vi "DJGUETTA.vi"() -> ()   [LabVIEW 2018]
uses:
  estadodjguetta.ctl
  <vilib>/myRIO/Express VI/Onboard IO/DI/DI Express VI.xnode
  <vilib>/myRIO/Instrument Drivers/Onboard IO/DIO/vis/Read.vi
  <vilib>/myRIO/Instrument Drivers/Onboard IO/DIO/DIO.lvlib
  <vilib>/myRIO/Common/Instrument Driver Framework/myRIO v1.0/DIO/typedefs/DIO Channels Enum.ctl
  <vilib>/myRIO/Common/Instrument Driver Framework/myRIO v1.0/DIO/typedefs/DIO Channels List.ctl
  <vilib>/myRIO/Common/Instrument Driver Framework/Utilities/typedefs/Generic FPGA Reference.ctl
  <vilib>/myRIO/Common/Instrument Driver Framework/Utilities/typedefs/myRIO v1.0 Reference.ctl
  <vilib>/myRIO/Common/Instrument Driver Framework/Utilities/typedefs/Hardware Version Enum.ctl
  <vilib>/myRIO/Common/Instrument Driver Framework/Utilities/typedefs/myRIO Generic Hardware Reference.ctl
  <vilib>/myRIO/Instrument Drivers/Onboard IO/DIO/typedefs/DIO Reference.ctl
  <vilib>/myRIO/Instrument Drivers/Onboard IO/DIO/vis/myRIO DIO Open.xnode
  <vilib>/myRIO/Common/Instrument Driver Framework/Utilities/vis/Is FPGA Ref Available.vi
  <vilib>/myRIO/Common/Instrument Driver Framework/myRIO v1.0/DIO/vis/myRIO v1.1 Open DIO.vi
  <vilib>/userdefined/High Color/nirio_resource_hc.ctl
panel:
  out "discos":i32
  out "yf":i32
  out "xf":i32
  out "Discos colocados":i32[](array[numeric])
  in  "Pieza":i32(slide) scale=0.0..2.0
  out "PteVertical":i32
  out "PteHH":i32
  out "Edos":T1
  in  "Start":bool
  out "Pulsos Vertical":i32
  out "Pulsos Horizontal":i32
  in  "stop":bool
  in  "Vertical":bool
  in  "Horizontal":bool
  # "Colocados en A\n\nColocados en B\n\nColocados en C"
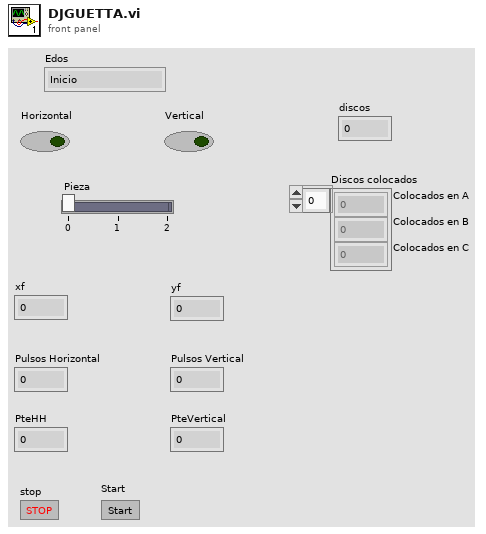
[diagram p1: front panel]
types:
  T1 = typedef "estadodjguetta.ctl" = enum16{"Inicio", "Baja1", "Pausa1", "Sube1", "Pausa2", "Derecha", "Pausa3", "Baja2", "Pausa4", "Sube2", "Pausa5", "Izq", "Pausa6", "Fin"}
  T2 = typedef "DIO.lvlib/DIO Reference.ctl" = cluster{"myRIO Reference":T3, "DIO Channels List":T7}
  T3 = typedef "myRIO Generic Hardware Reference.ctl" = cluster{"myRIO Model":T4, "myRIO Hardware Reference":T5}
  T4 = typedef "Hardware Version Enum.ctl" = enum16{"Unknown", "myRIO-1900", "myRIO-1950", "roboRIO", "NI ELVIS RIO CM", "ELVIS III"}
  T5 = typedef "myRIO v1.0 Reference.ctl" = cluster{"Generic FPGA Reference":T6, "Allow multiple opens":bool}
  T6 = typedef "Generic FPGA Reference.ctl" = refnum<k20>
  T7 = typedef "DIO Channels List.ctl" = T8[]
  T8 = typedef "DIO Channels Enum.ctl" = enum16{"Not Connected", "C/DIO0", "C/DIO1", "C/DIO2", "C/DIO3", "C/DIO4", "C/DIO5", "C/DIO6", "C/DIO7", "A/DIO0", "A/DIO1", "A/DIO2", "A/DIO3", "A/DIO4", "A/DIO5", "A/DIO6", "A/DIO7", "A/DIO8", "A/DIO9", "A/DIO10", "A/DIO11", "A/DIO12", "A/DIO13", "A/DIO14", "A/DIO15", "A/DIO16", "A/DIO17", "A/DIO18", "A/DIO19", "B/DIO0", "B/DIO1", "B/DIO2", "B/DIO3", "B/DIO4", "B/DIO5", "B/DIO6", "B/DIO7", "B/DIO8", "B/DIO9", "B/DIO10", "B/DIO11", "B/DIO12", "B/DIO13", "B/DIO14", "B/DIO15", "B/DIO16", "B/DIO17", "B/DIO18", "B/DIO19", "LED0", "LED1", "LED2", "LED3", "Button0", "DIO/DIO0", "DIO/DIO1", "DIO/DIO2", "DIO/DIO3", "DIO/DIO4", "DIO/DIO5", "DIO/DIO6", "DIO/DIO7", "DIO/DIO8", "DIO/DIO9", "SPI/CS0", "SPI/CS1", "SPI/CS2", "SPI/CS3", "LED RADIO (Green)", "LED RADIO (Red)", "LED COMM (Green)", "LED COMM (Red)", "LED MODE (Green)", "LED MODE (Red)"}
  T9 = typedef "nirio_resource_hc.ctl" = tag
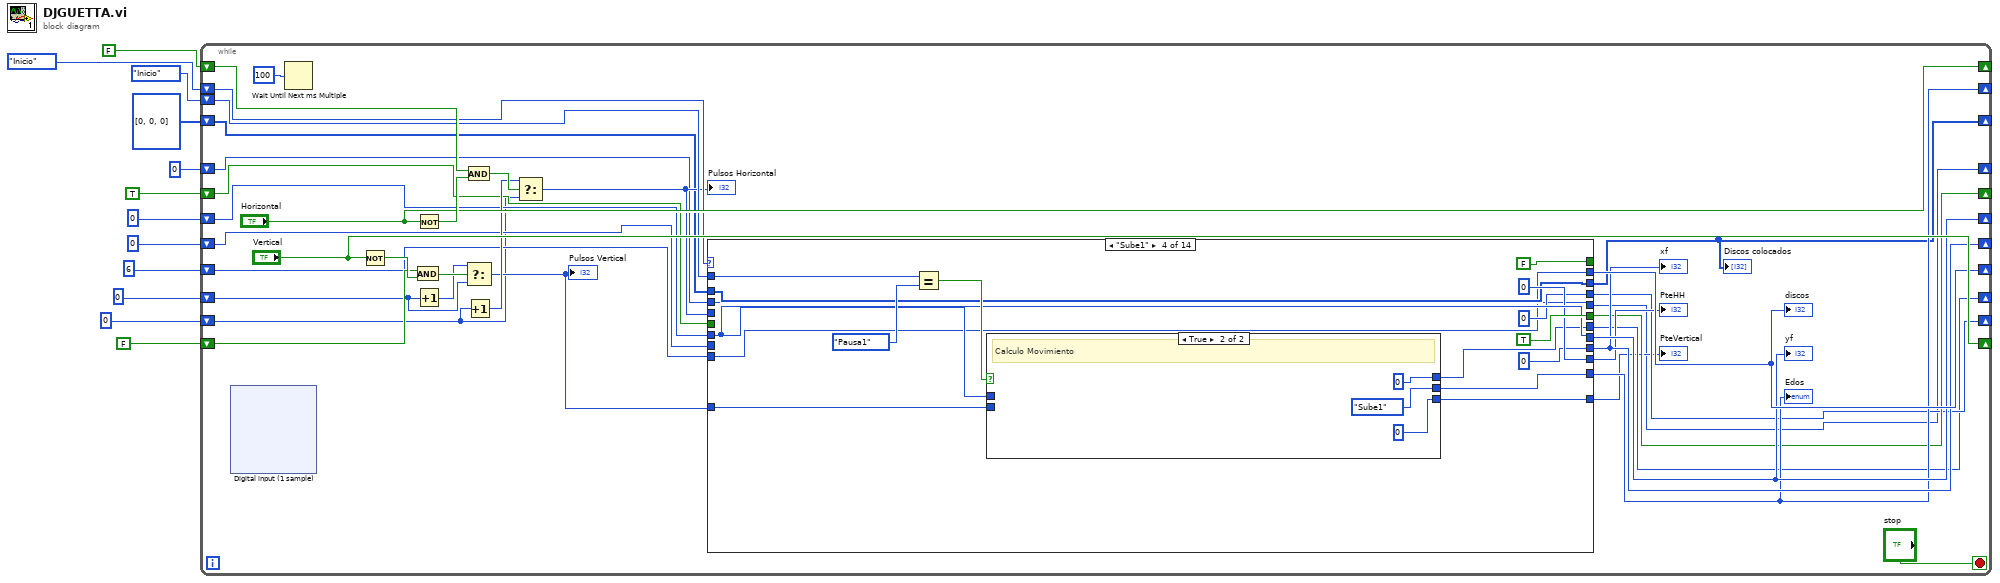
[diagram p0: block diagram]
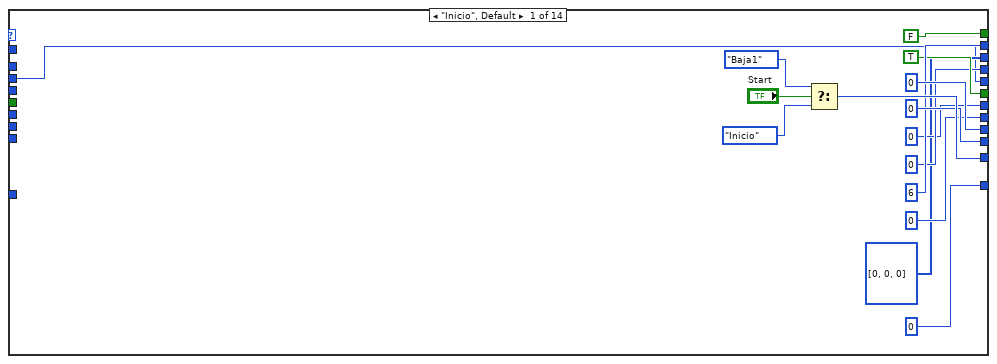
[diagram p2: hidden frame]
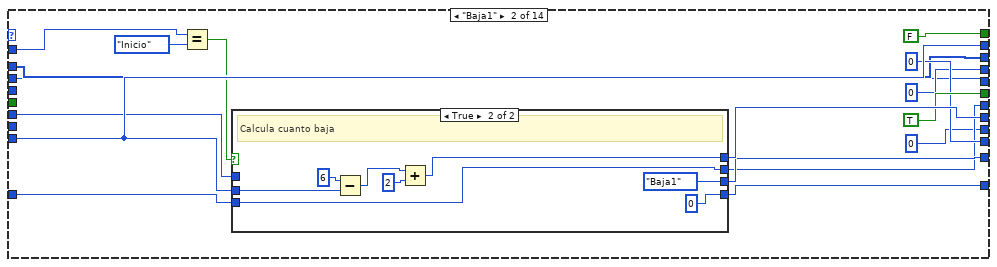
[diagram p3: hidden frame]
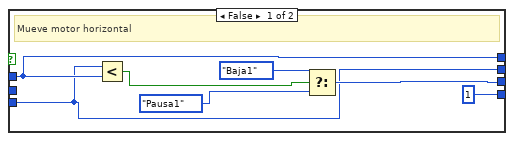
[diagram p4: hidden frame]
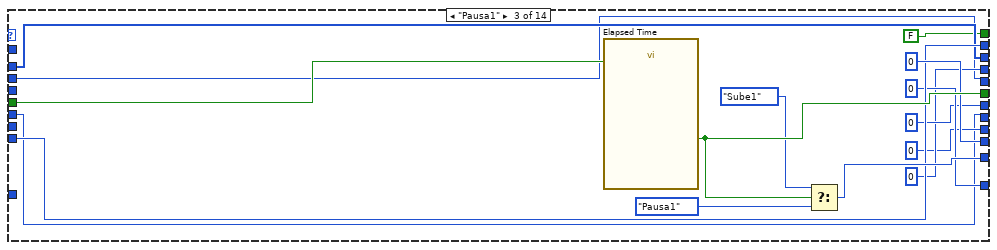
[diagram p5: hidden frame]
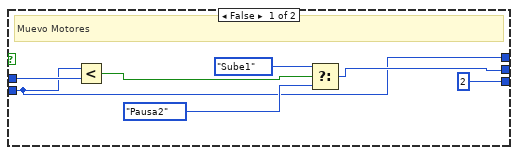
[diagram p6: hidden frame]
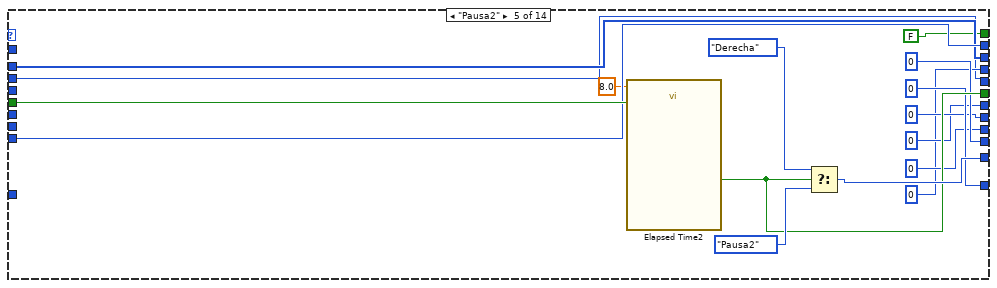
[diagram p7: hidden frame]
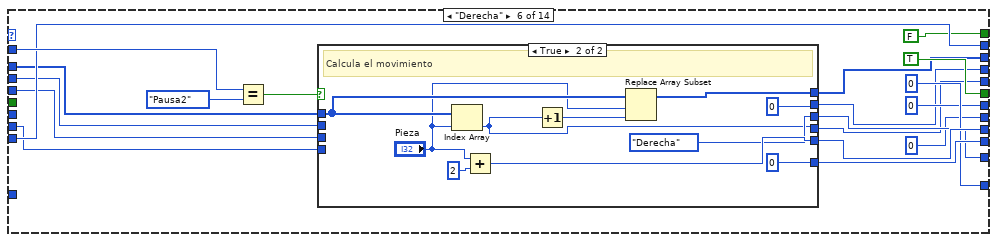
[diagram p8: hidden frame]
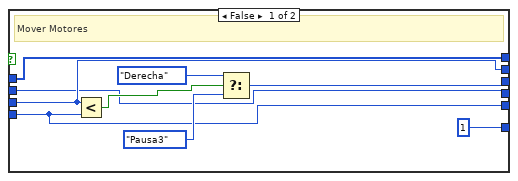
[diagram p9: hidden frame]
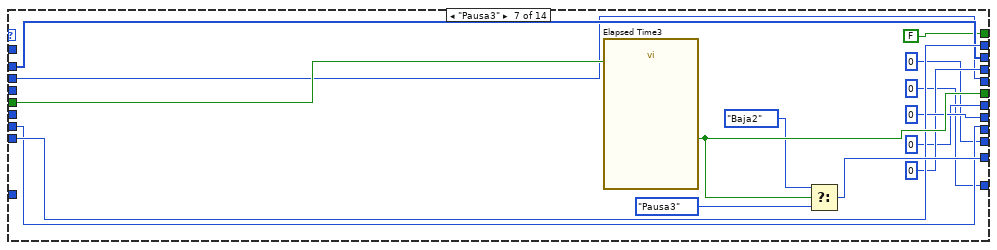
[diagram p10: hidden frame]
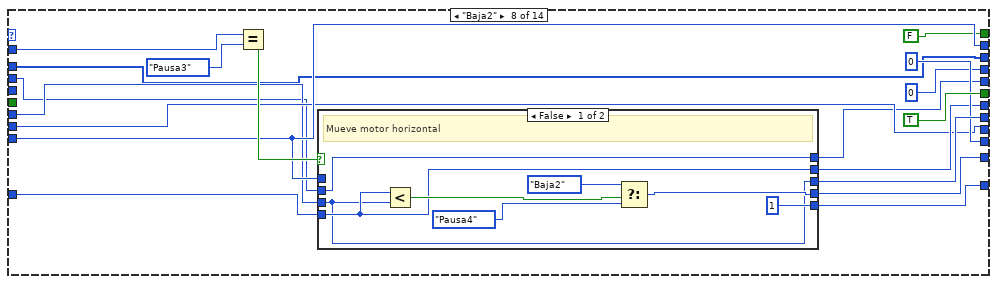
[diagram p11: hidden frame]
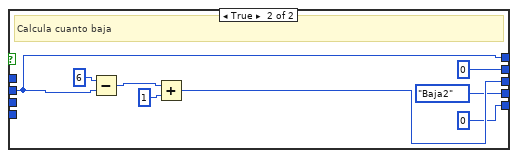
[diagram p12: hidden frame]
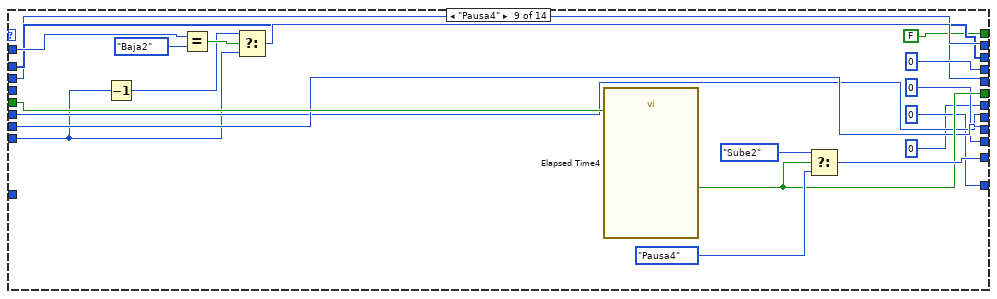
[diagram p13: hidden frame]
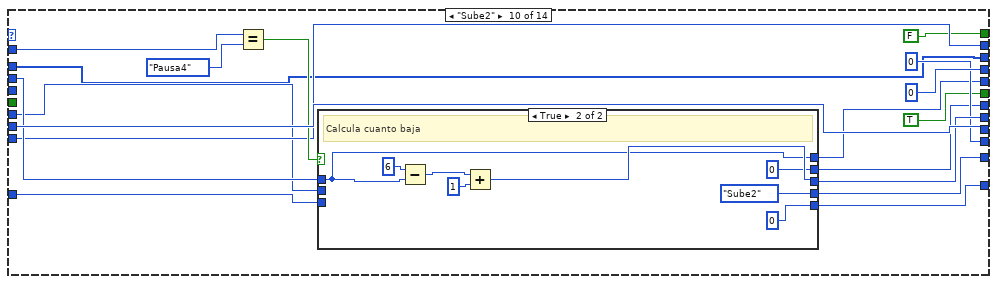
[diagram p14: hidden frame]
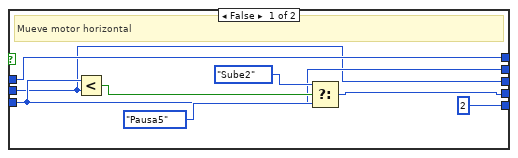
[diagram p15: hidden frame]
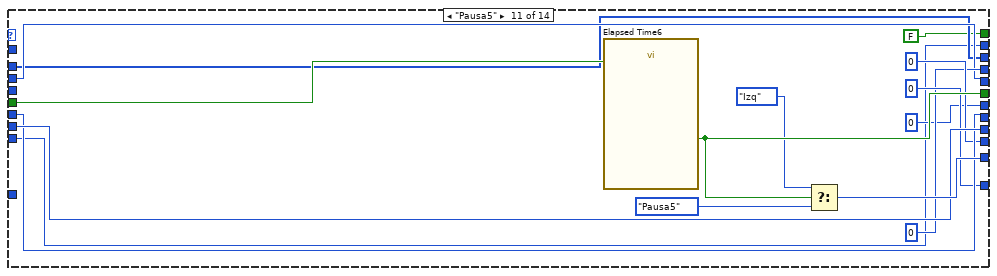
[diagram p16: hidden frame]
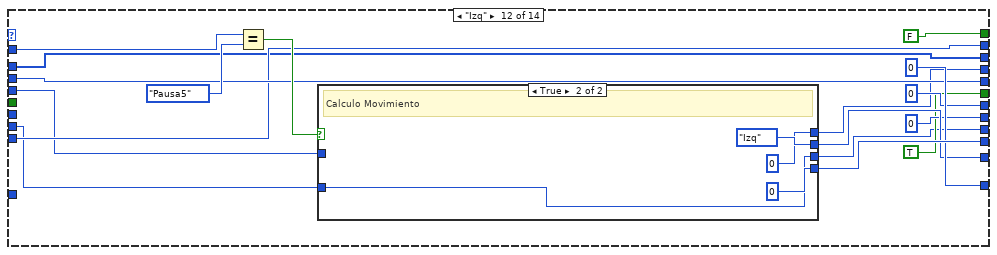
[diagram p17: hidden frame]
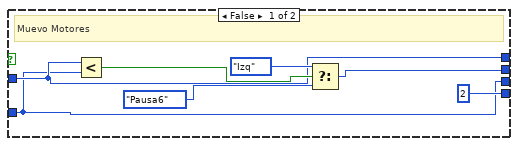
[diagram p18: hidden frame]
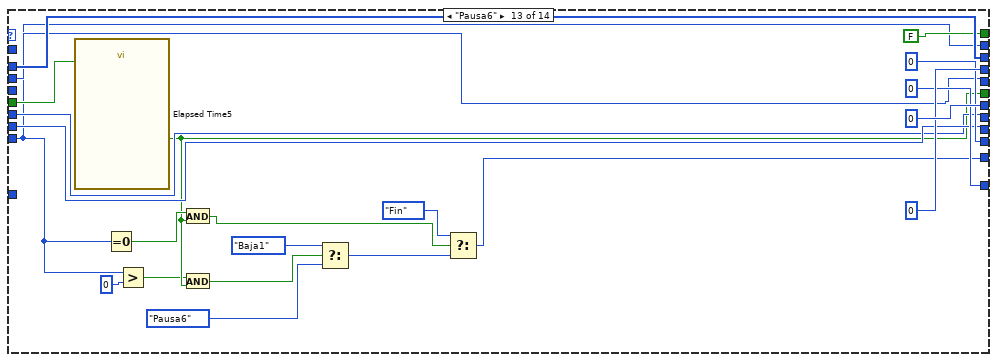
[diagram p19: hidden frame]
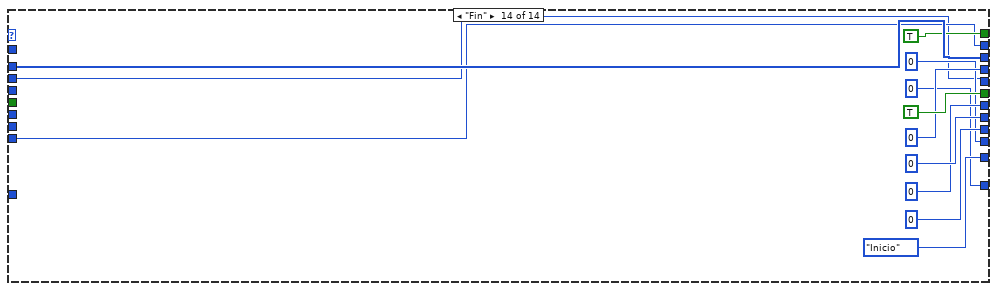
[diagram p20: hidden frame]
diagram:
  n1 = while {
    shift-right: ["Horizontal"] -> _
    shift-left: FALSE -> [w45]
    shift-right: ["Vertical"] -> _
    shift-left: FALSE -> [w43]
    shift-right: [w21] -> _
    shift-left: 0 -> [w22]
    shift-right: [w19] -> _
    shift-left: 0 -> [w36]
    shift-right: [w28] -> _
    shift-left: estadodjguetta."Inicio" -> [w35]
    shift-right: [w33] -> _
    shift-left: 6 -> [w34]
    shift-right: [w29] -> _
    shift-left: 0 -> [w30]
    shift-right: [w31] -> _
    shift-left: 0 -> [w32]
    shift-left: estadodjguetta."Inicio" -> [w27]
    shift-right: [w23] -> _
    shift-left: TRUE -> [w24]
    shift-right: [w16] -> _
    shift-left: i32[] [0, 0, 0] ("Discos colocados") -> [w17]
    shift-right: [w15] -> _
    shift-left: 0 -> [w14]
    stop <- "stop" stop-if-true
    n2 = xnode "Digital input (1 sample)"() -> ()  [unwired: 1 in, 2 out]
    n3 = Wait Until Next ms Multiple(millisecond multiple=100) -> ()  [unwired: 1 out]
    n4 = Not(x="Vertical") -> (.not. x?=w44:bool)
    n5 = And(x=w43, y=w44) -> (x .and. y?=w38:bool)
    n6 = Not(x="Horizontal") -> (.not. x?=w46:bool)
    n7 = Increment(x=w36) -> (x+1=w37:i32)
    n8 = And(x=w45, y=w46) -> (x .and. y?=w40:bool)
    n9 = Select(t=w37, s=w38, f=w36) -> (s? t:f=w26:i32)
    "Pulsos Vertical" <- w26
    n10 = Increment(x=w22) -> (x+1=w39:i32)
    n11 = Select(t=w39, s=w40, f=w22) -> (s? t:f=w20:i32)
    "Pulsos Horizontal" <- w20
    n12 = case shown="\"Sube1\"" w35 {
      tunnel: w34 -> [_ w112 w138 w145 w179 w195 w234 w250 w278 w304 w328 w350 w379 w398]
      tunnel: [6 w112 w138 w145 w179 w195 w234 w250 w277 w304 w328 w350 w379 w398] -> w33
      tunnel: w32 -> [_ w110 w133 w154 _ _ _ w246 w287 w297 w336 _ w386 _]
      tunnel: [0 w113 w133 w154 0 0 0 w254 w287 w305 w336 0 w386 0] -> w31
      tunnel: w30 -> [_ _ _ _ _ w192 w232 w247 w288 w311 w337 w347 w387 _]
      tunnel: [0 0 0 0 0 w202 w232 w247 w288 w311 w337 w343 w387 0] -> w29
      tunnel: [w94 w111 w140 w157 w184 w199 w235 w251 w290 w302 w338 w352 w371 estadodjguetta."Inicio"] -> w28
      tunnel: w27 -> [_ w103 _ w159 _ w205 _ w255 w282 w308 _ w356 _ _]
      tunnel: w26 -> [_ w109 _ w155 _ _ _ w248 _ w298 _ _ _ _]
      tunnel: [0 0 0 0 0 w201 0 0 0 0 0 w355 0 0] -> w25
      tunnel: w24 -> [_ _ w144 _ w183 _ w239 _ w293 _ w342 _ w392 _]
      tunnel: [TRUE TRUE w143 TRUE w182 TRUE w238 TRUE w289 TRUE w341 TRUE w377 TRUE] -> w23
      tunnel: [0 0 0 0 0 w196 0 0 0 0 0 w345 0 0] -> w21
      tunnel: w20 -> [_ _ _ _ _ w193 _ _ _ _ _ w346 _ _]
      tunnel: [0 w105 0 w151 0 0 0 w249 0 w299 0 0 0 0] -> w19
      tunnel: [0 w107 0 w153 0 0 0 w240 0 w306 0 0 0 0] -> w18
      tunnel: [i32[] [0, 0, 0] ("Discos colocados") w102 w132 w149 w174 w189 w227 w243 w276 w294 w330 w344 w385 w404] -> w16
      tunnel: w17 -> [_ w102 w132 w149 w174 w191 w227 w243 w276 w294 w330 w344 w385 w404]
      tunnel: [w83 w99 w130 w146 w171 w190 w225 w241 w274 w300 w331 w353 w383 w393] -> w15
      tunnel: w14 -> [w83 w99 w130 w146 w171 w187 w225 w244 w274 w307 w331 w353 w383 w393]
      tunnel: [FALSE FALSE FALSE FALSE FALSE FALSE FALSE FALSE FALSE FALSE FALSE FALSE FALSE TRUE] -> _
      frame "Inicio", Default {
        n13 = Select(t=estadodjguetta."Baja1", s="Start", f=estadodjguetta."Inicio") -> (s? t:f=w94:T1)
      }
      frame "Baja1" {
        n14 = Equal?(x=w103, y=estadodjguetta."Inicio") -> (x = y?=w98:bool)
        n15 = case shown="True" w98 {
          tunnel: w112 -> [_ w128]
          tunnel: [w116 w125] -> w113
          tunnel: [w118 estadodjguetta."Baja1" ("y")] -> w111
          tunnel: w110 -> [w116 _]
          tunnel: w109 -> [w115 w122]
          tunnel: [1 0] -> w107
          tunnel: [w115 w122] -> w105
          frame False {
            # "Mueve motor horizontal"
            n16 = Less?(x=w115, y=w116) -> (x < y?=w121:bool)
            n17 = Select(t=estadodjguetta."Baja1", s=w121, f=estadodjguetta."Pausa1") -> (s? t:f=w118:T1)
          }
          frame True {
            # "Calcula cuanto baja"
            n18 = Subtract(x=6, y=w128) -> (x-y=w127:i32)
            n19 = Add(x=w127, y=2) -> (x+y=w125:i32)
          }
        }
      }
      frame "Pausa1" {
        n20 = call "Elapsed Time"("Reset"=w144) -> ("Time has Elapsed"=w143:bool)  [unwired: 11 in, 7 out]
        n21 = Select(t=estadodjguetta."Sube1", s=w143, f=estadodjguetta."Pausa1") -> (s? t:f=w140:T1)
      }
      frame "Sube1" {
        n22 = Equal?(x=w159, y=estadodjguetta."Pausa1") -> (x = y?=w160:bool)
        n23 = case shown="True" w160 {
          tunnel: [2 0] -> w153
          tunnel: [w163 estadodjguetta."Sube1"] -> w157
          tunnel: [w162 0] -> w151
          tunnel: w155 -> [w162 _]
          tunnel: w154 -> [w167 _]
          frame False {
            # "Muevo Motores"
            n24 = Less?(x=w162, y=w167) -> (x < y?=w166:bool)
            n25 = Select(t=estadodjguetta."Sube1", s=w166, f=estadodjguetta."Pausa2") -> (s? t:f=w163:T1)
          }
          frame True {
            # "Calculo Movimiento"
          }
        }
      }
      frame "Pausa2" {
        n26 = call "Elapsed Time2"("Time Target (s)"=8.0, "Reset"=w183) -> ("Time has Elapsed"=w182:bool)  [unwired: 10 in, 7 out]
        n27 = Select(t=estadodjguetta."Derecha", s=w182, f=estadodjguetta."Pausa2") -> (s? t:f=w184:T1)
      }
      frame "Derecha" {
        n28 = Equal?(x=w205, y=estadodjguetta."Pausa2") -> (x = y?=w203:bool)
        n29 = case shown="True" w203 {
          tunnel: [w208 w223] -> w202
          tunnel: [1 0] -> w201
          tunnel: [w211 estadodjguetta."Derecha"] -> w199
          tunnel: [w210 0] -> w196
          tunnel: w193 -> [w210 _]
          tunnel: w192 -> [w208 _]
          tunnel: w191 -> [w206 w219]
          tunnel: [w207 w217] -> w190
          tunnel: [w206 w215] -> w189
          tunnel: w187 -> [w207 _]
          frame False {
            # "Mover Motores"
            n30 = Less?(x=w210, y=w208) -> (x < y?=w214:bool)
            n31 = Select(t=estadodjguetta."Derecha", s=w214, f=estadodjguetta."Pausa3") -> (s? t:f=w211:T1)
          }
          frame True {
            # "Calcula el movimiento"
            n32 = Index Array(array=w219, index="Pieza") -> (element=w217:i32)
            n33 = Add(x="Pieza", y=2) -> (x+y=w223:i32)
            n34 = Increment(x=w217) -> (x+1=w216:i32)
            n35 = Replace Array Subset(array=w219, new element=w216, index="Pieza") -> (w215:i32[])
          }
        }
      }
      frame "Pausa3" {
        n36 = call "Elapsed Time3"("Reset"=w239) -> ("Time has Elapsed"=w238:bool)  [unwired: 11 in, 7 out]
        n37 = Select(t=estadodjguetta."Baja2", s=w238, f=estadodjguetta."Pausa3") -> (s? t:f=w235:T1)
      }
      frame "Baja2" {
        n38 = Equal?(x=w255, y=estadodjguetta."Pausa3") -> (x = y?=w257:bool)
        n39 = case shown="False" w257 {
          tunnel: [w259 w270] -> w254
          tunnel: [w262 estadodjguetta."Baja2" ("y")] -> w251
          tunnel: [1 0] -> w240
          tunnel: w250 -> [_ _]
          tunnel: [w260 0] -> w249
          tunnel: w248 -> [w260 _]
          tunnel: w246 -> [w259 _]
          tunnel: w244 -> [w258 w266]
          tunnel: [w258 w266] -> w241
          frame False {
            # "Mueve motor horizontal"
            n40 = Less?(x=w260, y=w259) -> (x < y?=w265:bool)
            n41 = Select(t=estadodjguetta."Baja2", s=w265, f=estadodjguetta."Pausa4") -> (s? t:f=w262:T1)
          }
          frame True {
            # "Calcula cuanto baja"
            n42 = Subtract(x=6, y=w266) -> (x-y=w272:i32)
            n43 = Add(x=w272, y=1) -> (x+y=w270:i32)
          }
        }
      }
      frame "Pausa4" {
        n44 = Decrement(x=w278) -> (x-1=w279:i32)
        n45 = Equal?(x=w282, y=estadodjguetta."Baja2") -> (x = y?=w280:bool)
        n46 = Select(t=w279, s=w280, f=w278) -> (s? t:f=w277:i32)
        n47 = call "Elapsed Time4"("Reset"=w293) -> ("Time has Elapsed"=w289:bool)  [unwired: 11 in, 7 out]
        n48 = Select(t=estadodjguetta."Sube2", s=w289, f=estadodjguetta."Pausa4") -> (s? t:f=w290:T1)
      }
      frame "Sube2" {
        n49 = Equal?(x=w308, y=estadodjguetta."Pausa4") -> (x = y?=w310:bool)
        n50 = case shown="True" w310 {
          tunnel: [w312 w324] -> w305
          tunnel: [w316 estadodjguetta."Sube2" ("y")] -> w302
          tunnel: [w314 0] -> w299
          tunnel: [2 0] -> w306
          tunnel: w307 -> [w313 w320]
          tunnel: [w313 w320] -> w300
          tunnel: w298 -> [w314 _]
          tunnel: w297 -> [w312 _]
          frame False {
            # "Mueve motor horizontal"
            n51 = Less?(x=w314, y=w312) -> (x < y?=w319:bool)
            n52 = Select(t=estadodjguetta."Sube2", s=w319, f=estadodjguetta."Pausa5") -> (s? t:f=w316:T1)
          }
          frame True {
            # "Calcula cuanto baja"
            n53 = Subtract(x=6, y=w320) -> (x-y=w326:i32)
            n54 = Add(x=w326, y=1) -> (x+y=w324:i32)
          }
        }
      }
      frame "Pausa5" {
        n55 = call "Elapsed Time6"("Reset"=w342) -> ("Time has Elapsed"=w341:bool)  [unwired: 11 in, 7 out]
        n56 = Select(t=estadodjguetta."Izq", s=w341, f=estadodjguetta."Pausa5") -> (s? t:f=w338:T1)
      }
      frame "Izq" {
        n57 = Equal?(x=w356, y=estadodjguetta."Pausa5") -> (x = y?=w358:bool)
        n58 = case shown="True" w358 {
          tunnel: [w363 estadodjguetta."Izq"] -> w352
          tunnel: [2 0] -> w355
          tunnel: w347 -> [w360 w367]
          tunnel: w346 -> [w361 _]
          tunnel: [w361 0] -> w345
          tunnel: [w360 w367] -> w343
          frame False {
            # "Muevo Motores"
            n59 = Less?(x=w361, y=w360) -> (x < y?=w366:bool)
            n60 = Select(t=estadodjguetta."Izq", s=w366, f=estadodjguetta."Pausa6") -> (s? t:f=w363:T1)
          }
          frame True {
            # "Calculo Movimiento"
          }
        }
      }
      frame "Pausa6" {
        n61 = call "Elapsed Time5"("Reset"=w392) -> ("Time has Elapsed"=w377:bool)  [unwired: 11 in, 7 out]
        n62 = Equal To 0?(x=w379) -> (x = 0?=w382:bool)
        n63 = Greater?(x=w379, y=0) -> (0:w376:bool)
        n64 = And(x=w382, y=w377) -> (x .and. y?=w381:bool)
        n65 = And(x=w376, y=w377) -> (x .and. y?=w375:bool)
        n66 = Select(t=estadodjguetta."Baja1", s=w375, f=estadodjguetta."Pausa6") -> (s? t:f=w372:T1)
        n67 = Select(t=estadodjguetta."Fin", s=w381, f=w372) -> (s? t:f=w371:T1)
      }
      frame "Fin" {
      }
    }
    "Edos" <- w28
    "PteHH" <- w25
    "PteVertical" <- w18
    "Discos colocados" <- w16
    "xf" <- w29
    "yf" <- w31
    "discos" <- w33
  }
